vi "判断是否为数字字符串.vi"(1 "字符串":string) -> (0 "是否为数字":bool)   [LabVIEW 2014]
doc: "该模板用于创建子VI。"
panel:
  out "error out":errorcluster caption="错误输出"
  in  "error in (no error)":errorcluster caption="错误输入（无错误）"
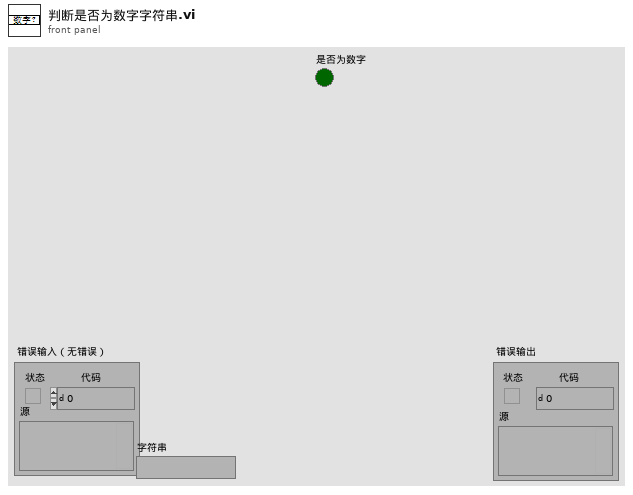
[diagram p1: front panel]
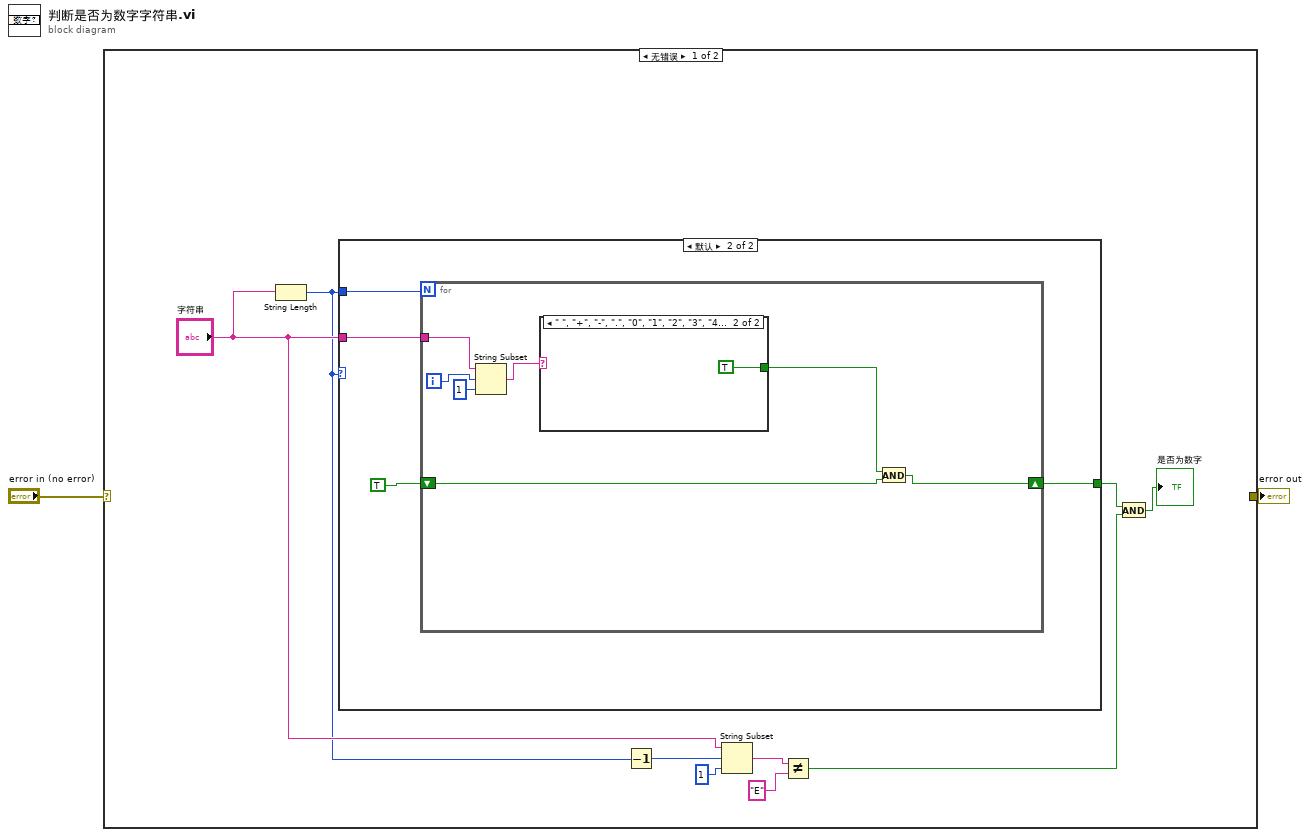
[diagram p0: block diagram]
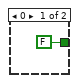
[diagram p2: hidden frame]
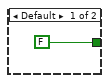
[diagram p3: hidden frame]
diagram:
  n1 = case shown="无错误" "error in (no error)" {
    selector: "error in (no error)" -> [_ w26]
    tunnel: [_ w26] -> w1
    frame No Error {
      n2 = String Length(string="字符串") -> (length=w10:i32)
      n3 = case shown="默认" w10 {
        tunnel: w10 -> [_ w16]
        tunnel: "字符串" -> [_ w15]
        tunnel: [FALSE w13] -> w5
        frame 0 {
        }
        frame Default {
          n4 = for {
            N: w16 -> [_]
            tunnel: w15 -> [w22]
            shift-right: [w17] -> w13
            shift-left: TRUE -> [w18]
            i -> [w21]
            n5 = String Subset(string=w22, offset (0)=w21, length (rest)=1 ("长度（剩余）")) -> (substring=w20:string)
            n6 = case shown="\" \", \"+\", \"-\", \".\", \"0\", \"1\", \"2\", \"3\", \"4\", \"5\", \"6\", \"7\", \"8\", \"9\", \"E\", \"e\"" w20 {
              tunnel: [FALSE TRUE] -> w19
              frame Default {
              }
              frame " ", "+", "-", ".", "0", "1", "2", "3", "4", "5", "6", "7", "8", "9", "E", "e" {
              }
            }
            n7 = And(x=w19, y=w18) -> (x .and. y?=w17:bool)
          }
        }
      }
      n8 = Decrement(x=w10) -> (x-1=w9:i32)
      n9 = String Subset(string="字符串", offset (0)=w9, length (rest)=1 ("长度（剩余）")) -> (substring=w7:string)
      n10 = Not Equal?(x=w7, y="E") -> (x != y?=w4:bool)
      n11 = And(x=w5, y=w4) -> (x .and. y?=→"是否为数字":bool)
    }
    frame Error {
    }
  }
  "error out" <- w1
